vi "Module Type.vi"(11 "Telemetry Server Module in":refnum<class "Telemetry Server Module.lvclass">) -> (2 "Module Type":string)   [LabVIEW 2020, in "Volatus.lvlib" / "Telemetry Server Module.lvclass"]
uses:
  Telemetry Server Module.lvclass
  Telemetry Server Module.lvclass/Telemetry Server Module.ctl
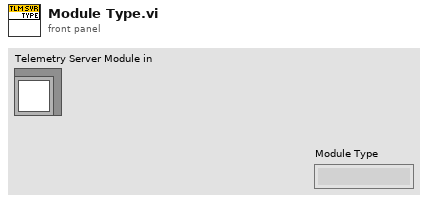
[diagram p1: front panel]
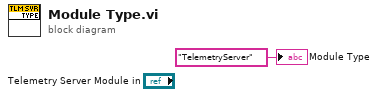
[diagram p0: block diagram]
diagram:
  "Module Type" <- "TelemetryServer" ("Module Type")
